vi "DETStatus-Com-Exec.vi"(8 "error in (no error)":errorcluster, 11 "DAQmxTaskContainer in":refnum<class "DAQmxTaskContainer.lvclass">) -> (0 "error out":errorcluster, 3 "DAQmxTaskContainer out":refnum<class "DAQmxTaskContainer.lvclass">)   [LabVIEW 2015, in "DAQmxTaskContainer.lvclass"]
uses:
  DAQmxTaskContainer/DAQmxTaskContainer.lvclass
  DAQmxTask.lvclass
  dependecies/ControlsVIs/Clusters-def/DAQmx-Reply-Connect-client.ctl
  DAQmxTaksContainer_General.lvclass
  Message/Message.lvclass
  dependecies/ControlsVIs/Clusters-def/SERVER-Commands.ctl
  Control/Control-Server/Control-Server.lvclass
  dependecies/ControlsVIs/Clusters-def/Message types.ctl
  GeneralFunctionality/GeneralFunctionality.lvclass
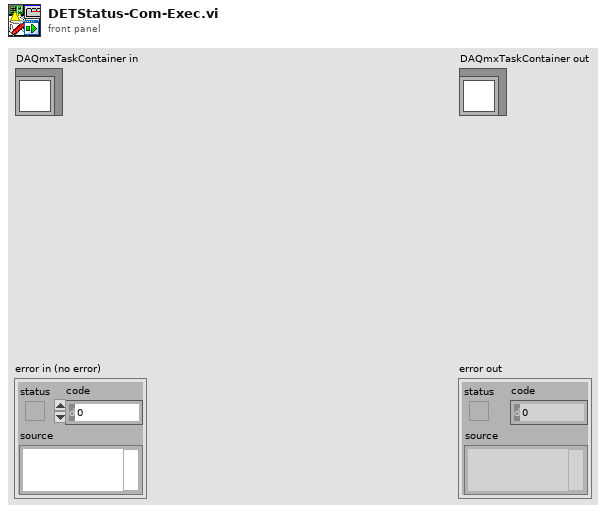
[diagram p1: front panel]
types:
  T1 = typedef "Message types.ctl" = string
  T2 = typedef "Control-Server.lvclass/SERVER-Commands.ctl" = string
  T3 = typedef "DAQmxTaksContainer_General.lvclass/DAQmx-Reply-Connect-client.ctl" = cluster{"on/off":bool, "RelayKeyHeater/off":bool, "LaserShutter":bool, "AcceleratorShutter":bool, "Power":bool, "Faraday Cup Status":bool, "error":errorcluster}
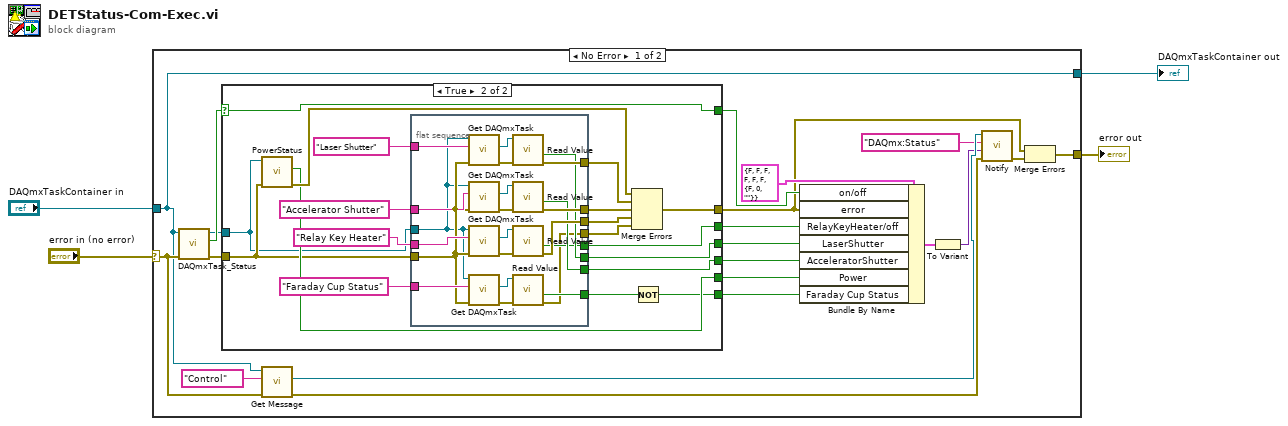
[diagram p0: block diagram]
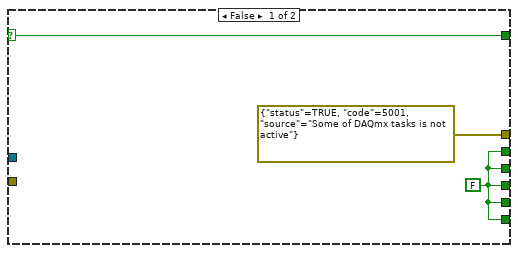
[diagram p2: hidden frame]
diagram:
  n1 = case shown="No Error" "error in (no error)" {
    selector: "error in (no error)" -> [w14 w71]
    tunnel: [w7 w71] -> w3
    tunnel: [w13 w70] -> w1
    tunnel: "DAQmxTaskContainer in" -> [w13 w70]
    frame No Error {
      n2 = call-dynamic "DAQmxTask_Status.vi"("error in (no error)"=w14, "DAQmxTaskContainer_General en entrée"=w13) -> ("error out"=w20:errorcluster, "All active"=w19:bool, "DAQmxTaskContainer_General en sortie"=w18:refnum<class "DAQmxTaskContainer.lvclass">)  [unwired: 6 in, 1 out]
      n3 = case shown="True" w19 {
        selector: w19 -> [w27 w35]
        tunnel: [errorcluster {"status"=TRUE, "code"=5001, "source"="Some of DAQmx tasks is not active"} ("error IO") w41] -> w16
        tunnel: [w26 w36] -> w21
        tunnel: [w26 w40] -> w22
        tunnel: [w26 w39] -> w23
        tunnel: [w26 w38] -> w24
        tunnel: w20 -> [_ w33]
        tunnel: w18 -> [_ w30]
        tunnel: [w27 w35] -> w17
        tunnel: [w26 w29] -> w5
        frame False {
          w26 = FALSE ("Data")
        }
        frame True {
          n4 = call "PowerStatus.vi"("error in (no error)"=w33, "DAQmxTaskContainer_General in"=w30) -> ("error out"=w37:errorcluster, "On/Off"=w36:bool)  [unwired: 7 in, 1 out]
          n5 = flat-sequence {
            tunnel: [w69] -> w47
            tunnel: [w68] -> w46
            tunnel: [w67] -> w45
            tunnel: "Relay Key Heater" ("Task name") -> [w60]
            tunnel: "Accelerator Shutter" ("Task name") -> [w59]
            tunnel: "Laser Shutter" ("Task name") -> [w58]
            tunnel: [w57] -> w40
            tunnel: [w56] -> w39
            tunnel: [w55] -> w38
            tunnel: "Faraday Cup Status" ("Task name") -> [w53]
            tunnel: w33 -> [w52]
            tunnel: [w51] -> w32
            tunnel: [w49] -> w31
            tunnel: w30 -> [w48]
            frame #0 {
              n6 = call "Get DAQmxTask.vi"("error in (no error)"=w52, "Task name"=w58, "DAQmxTaksContainer_General in"=w48) -> ("error out"=w61:errorcluster, "DAQmx Task"=w62:refnum<class "DAQmxTask.lvclass">)  [unwired: 6 in, 1 out]
              n7 = call "Get DAQmxTask.vi"("error in (no error)"=w52, "Task name"=w59, "DAQmxTaksContainer_General in"=w48) -> ("error out"=w63:errorcluster, "DAQmx Task"=w64:refnum<class "DAQmxTask.lvclass">)  [unwired: 6 in, 1 out]
              n8 = call "Get DAQmxTask.vi"("error in (no error)"=w52, "Task name"=w60, "DAQmxTaksContainer_General in"=w48) -> ("error out"=w65:errorcluster, "DAQmx Task"=w66:refnum<class "DAQmxTask.lvclass">)  [unwired: 6 in, 1 out]
              n9 = call "Get DAQmxTask.vi"("error in (no error)"=w52, "Task name"=w53, "DAQmxTaksContainer_General in"=w48) -> ("error out"=w50:errorcluster, "DAQmx Task"=w54:refnum<class "DAQmxTask.lvclass">)  [unwired: 6 in, 1 out]
              n10 = call-dynamic "Read Value.vi"("error in (no error)"=w61, "DAQmxTask en entrée"=w62) -> ("error out"=w67:errorcluster, "Data"=w57:bool)  [unwired: 6 in, 2 out]
              n11 = call-dynamic "Read Value.vi"("error in (no error)"=w63, "DAQmxTask en entrée"=w64) -> ("error out"=w68:errorcluster, "Data"=w56:bool)  [unwired: 6 in, 2 out]
              n12 = call-dynamic "Read Value.vi"("error in (no error)"=w65, "DAQmxTask en entrée"=w66) -> ("error out"=w69:errorcluster, "Data"=w55:bool)  [unwired: 6 in, 2 out]
              n13 = call-dynamic "Read Value.vi"("error in (no error)"=w50, "DAQmxTask en entrée"=w54) -> ("error out"=w49:errorcluster, "Data"=w51:bool)  [unwired: 6 in, 2 out]
            }
          }
          n14 = Merge Errors(w37, w45, w46, w47, w31) -> (w41:errorcluster)
          n15 = Not(x=w32) -> (.not. x?=w29:bool)
        }
      }
      n16 = call "Get Message.vi"("error in (no error)"=w14, "Message type"=T1 "Control", "GeneralFunctionality en entrée"=w13) -> ("error out"=w11:errorcluster, "Message.lvclass"=w12:refnum<class "Message.lvclass">)  [unwired: 6 in, 1 out]
      n17 = Bundle By Name(cluster=T3 {"on/off"=FALSE, "RelayKeyHeater/off"=FALSE, "LaserShutter"=FALSE, "AcceleratorShutter"=FALSE, "Power"=FALSE, "Faraday Cup Status"=FALSE, "error"={"status"=FALSE, "code"=0, "source"=""}} ("output cluster"), "on/off"=w17, "error"=w16, "RelayKeyHeater/off"=w24, "LaserShutter"=w22, "AcceleratorShutter"=w23, "Power"=w21, "Faraday Cup Status"=w5) -> (w15:T3)
      n18 = To Variant(anything=w15) -> (Variant=w10:variant)
      n19 = call "Notify.vi"("error in (no error)"=w11, "Data"=w10, "command"=T2 "DAQmx:Status" ("Commands"), "Message en entrée"=w12) -> ("error out"=w8:errorcluster)  [unwired: 6 in, 1 out]
      n20 = Merge Errors(w16, w8) -> (w7:errorcluster)
    }
    frame Error {
    }
  }
  "error out" <- w3
  "DAQmxTaskContainer out" <- w1
